vi "write Cell String to excel location.vi"(8 "error in (no error)":errorcluster, 9 "input string":string, 10 "cell's name":string, 11 "NI_report in":refnum<class "NI_report.lvclass">) -> (0 "error out":errorcluster, 3 "NI_report out":refnum<class "NI_report.lvclass">)   [LabVIEW 2016]
uses:
  <vilib>/Utility/NIReport.llb/NI_report.lvclass
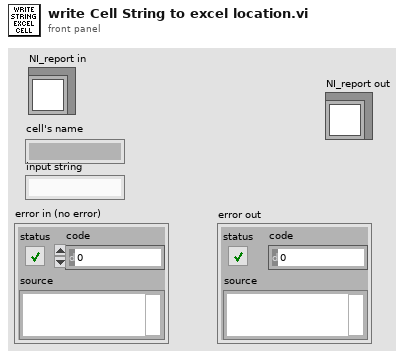
[diagram p1: front panel]
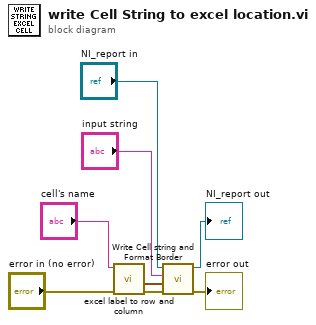
[diagram p0: block diagram]
diagram:
  n1 = call "excel label to row and column.vi"("error in (no error)"="error in (no error)", "cell's name"="cell's name") -> ("error IO"=w8:errorcluster, "output cluster"=w7:cluster{"row":i32, "column":i32})  [unwired: 5 in, 3 out]
  n2 = call "Write Cell string and Format Border.vi"("error in (no error)"=w8, "output cluster"=w7, "input string"="input string", "NI_report in"="NI_report in") -> ("error out"=→"error out":errorcluster, "NI_report out"=→"NI_report out":refnum<class "NI_report.lvclass">)  [unwired: 6 in]
